vi "Read Last Voltage.vi"(8 "error in (no error)":errorcluster, 10 "Channel":u8, 11 "Scope Base in":refnum<class "Scope Base.lvclass">) -> (0 "error out":errorcluster, 2 "Voltage":dbl, 3 "Scope Base out":refnum<class "Scope Base.lvclass">)   [LabVIEW 2023, in "Scope Base.lvlib" / "Scope Base.lvclass"]
uses:
  Scope Base.lvclass
  Scope Base.lvclass/Scope Base.ctl
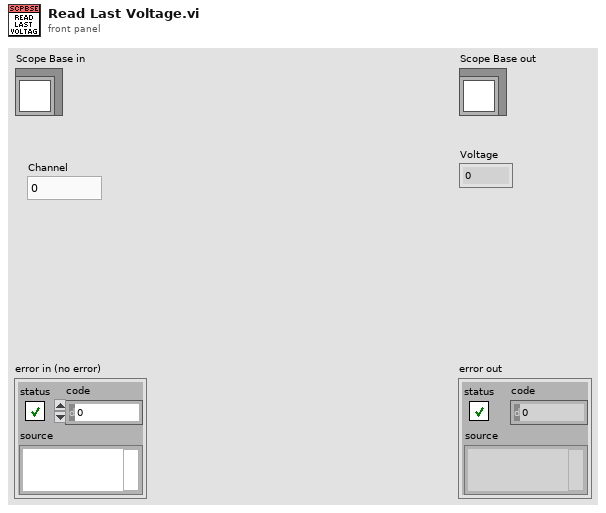
[diagram p1: front panel]
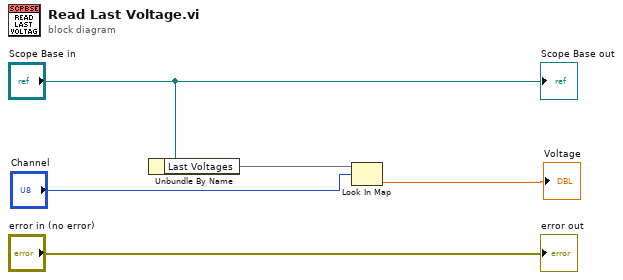
[diagram p0: block diagram]
diagram:
  n1 = Unbundle By Name("Scope Base in") -> ("Last Voltages"=w1:map{u8, dbl})
  n2 = Look In Map(map=w1, key="Channel") -> (value=→"Voltage":dbl)  [unwired: 1 in, 1 out]
  "error out" <- "error in (no error)"
  "Scope Base out" <- "Scope Base in"
